vi "GenerateHeaders.vi"(1 "Extra headers":string, 2 "UI Data":T1) -> (0 "Output headers":string)   [LabVIEW 2015]
uses:
  controls/UI Data.ctl
  controls/BridgeSettings.ctl
  Driver/Typedefs/OutputChannelTypedef.ctl
  controls/ChannelSelection.ctl
  Driver/Typedefs/InputChannelTypedef.ctl
  controls/ChannelSettings.ctl
  Driver/YbTempCtrl.lvlib
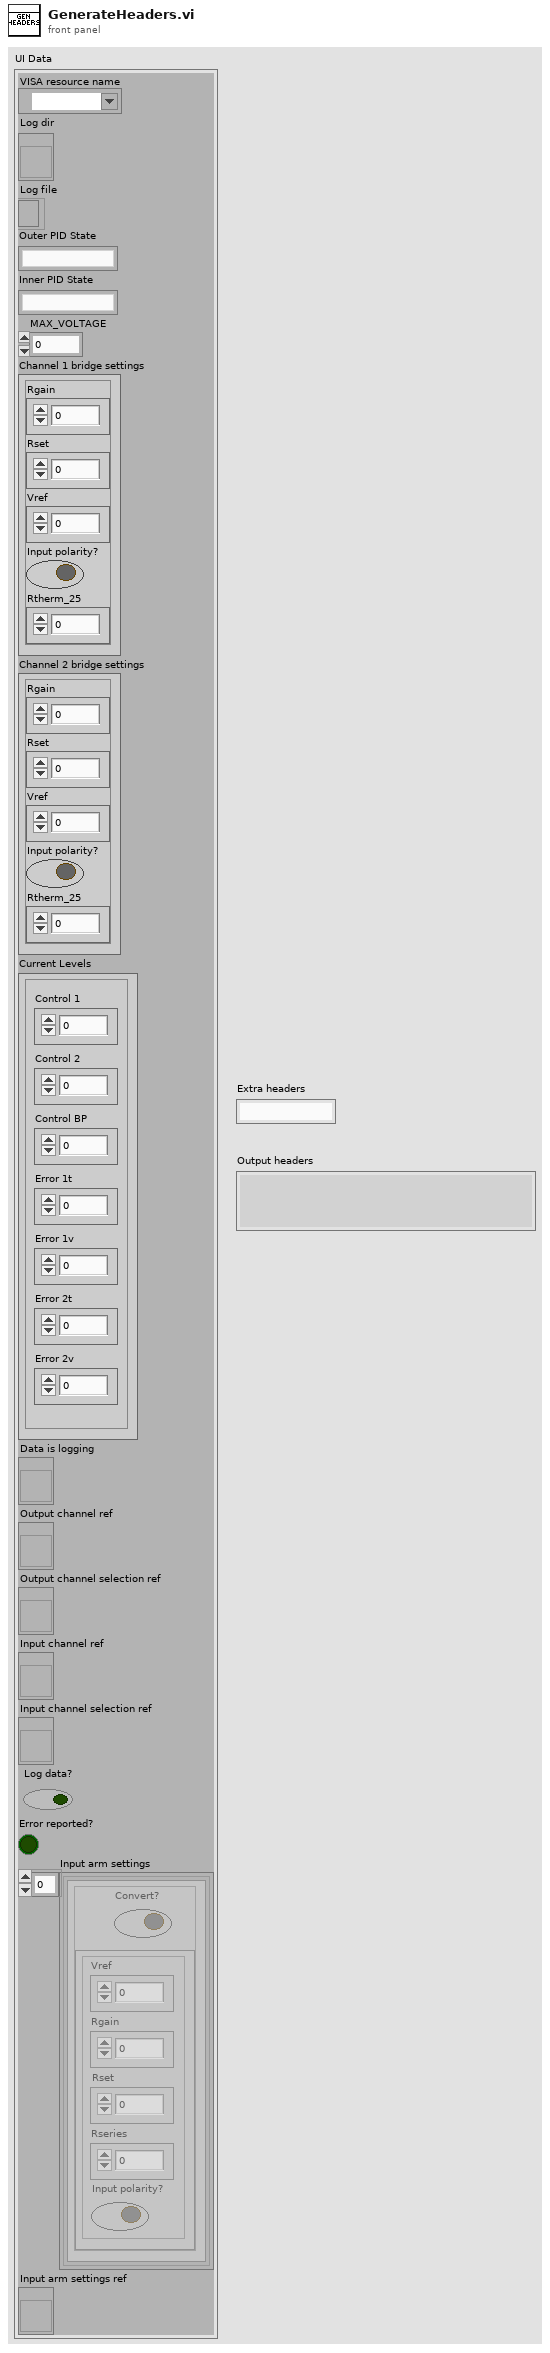
[diagram p1: front panel]
types:
  T1 = typedef "UI Data.ctl" = cluster{"VISA resource name":refnum<visa-resource-name>, "Log dir":refnum<vi>, "Log file":refnum<file>, "Outer PID State":string, "Inner PID State":string, "MAX_VOLTAGE":dbl, "Channel 1 bridge settings":T2, "Channel 2 bridge settings":T2, "Current Levels":cluster{"Control 1":dbl, "Control 2":dbl, "Control BP":dbl, "Error 1t":dbl, "Error 1v":dbl, "Error 2t":dbl, "Error 2v":dbl}, "Data is logging":refnum<vi>, "Output channel ref":refnum<vi>, "Output channel selection ref":refnum<vi>, "Input channel ref":refnum<vi>, "Input channel selection ref":refnum<vi>, "Log data?":bool, "Error reported?":bool, "Input arm settings":cluster{"Enum string":string, "Enum ID":i16, "Input arm settings":T3}[], "Input arm settings ref":refnum<vi>}
  T2 = typedef "BridgeSettings.ctl" = cluster{"Rgain":dbl, "Rset":dbl, "Vref":dbl, "Input polarity?":bool, "Rtherm_25":dbl}
  T3 = typedef "ChannelSettings.ctl" = cluster{"Convert?":bool, "Config":cluster{"Vref":dbl, "Rgain":dbl, "Rset":dbl, "Rseries":dbl, "Input polarity?":bool}}
  T4 = typedef "ChannelSelection.ctl" = cluster{"Channel name":string, "Enum id":u16, "Logging?":bool}[]
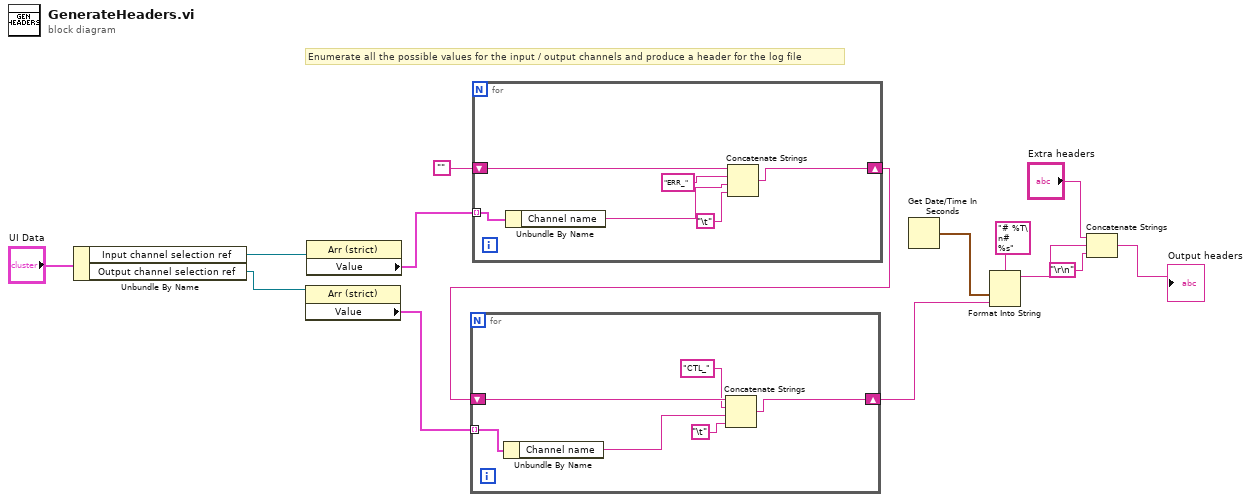
[diagram p0: block diagram]
diagram:
  # "Enumerate all the possible values for the input / output channels and produce a header for the log file"
  n1 = Unbundle By Name("UI Data") -> ("Input channel selection ref"=w13:refnum<vi>, "Output channel selection ref"=w12:refnum<vi>)
  n2 = property class="Arr (strict)"(reference=w12) -> ("Value"=w5:T4)  [unwired: 1 in, 2 out]
  n3 = property class="Arr (strict)"(reference=w13) -> ("Value"=w10:T4)  [unwired: 1 in, 2 out]
  n4 = for {
    shift-right: [w19] -> w6
    shift-left: "" -> [w20]
    tunnel: w10 -> [w18] mode=indexing
    n5 = Unbundle By Name(w18) -> ("Channel name"=w17:string)
    n6 = Concatenate Strings(w20, "ERR_", w17, "\t") -> (w19:string)
  }
  n7 = for {
    shift-right: [w25] -> w7
    shift-left: w6 -> [w26]
    tunnel: w5 -> [w23] mode=indexing
    n8 = Unbundle By Name(w23) -> ("Channel name"=w24:string)
    n9 = Concatenate Strings(w26, "CTL_", w24, "\t") -> (w25:string)
  }
  n10 = Get Date/Time In Seconds() -> (seconds since 1Jan1904=w8:timestamp)
  n11 = Format Into String(format string="# %T\n# %s", w8, w7) -> (resulting string=w4:string)  [unwired: 2 in, 1 out]
  n12 = Concatenate Strings("Extra headers", w4, "\r\n") -> (→"Output headers":string)
